vi "Progra 15.vi"() -> ()   [LabVIEW 2011]
uses:
  Control 2.ctl
  <vilib>/express/express arith-compare/Formula/XNode/ExpressFormulaBlockNode.xnode
panel:
  out "Array 2":string[](array[string])
  out "Array":dbl[](array[numeric])
  # "En el arreglo 1 ingresar 5 numeros enteros y luego en el arreglo 2\nescribir si es par o impar cada uno de los numeros"
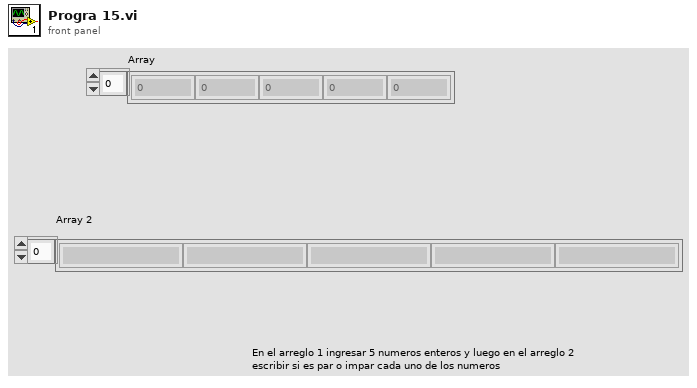
[diagram p1: front panel]
types:
  T1 = typedef "Control 2.ctl" = enum16{"Iniciar Arreglos", "Rellenar Arreglos", "Encontrar ParesImpares", "Final"}
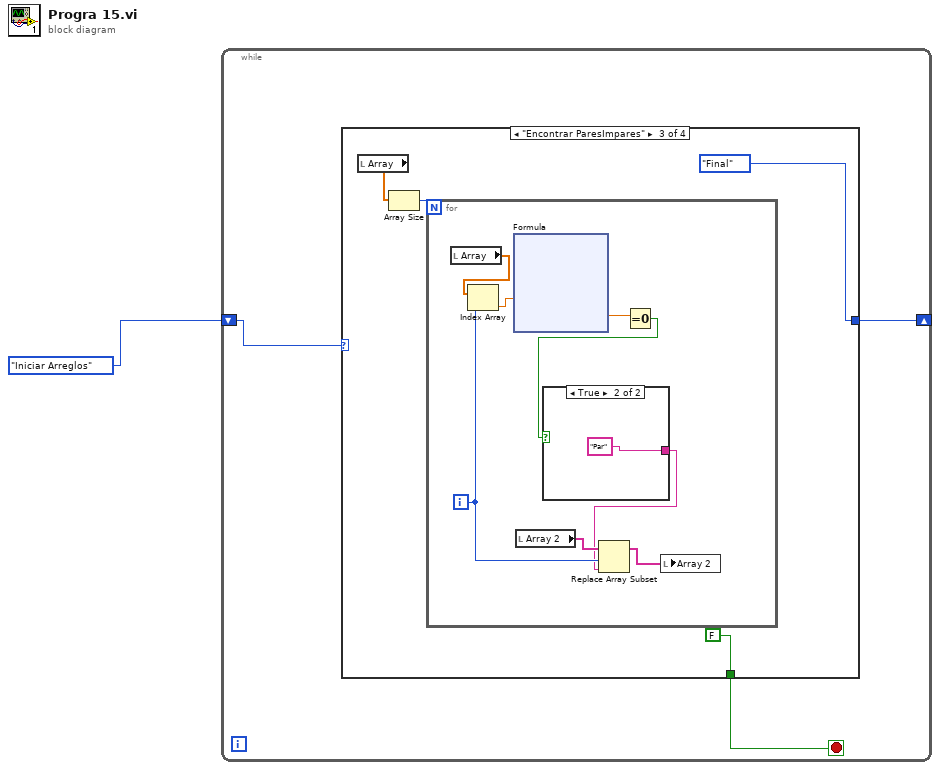
[diagram p0: block diagram]
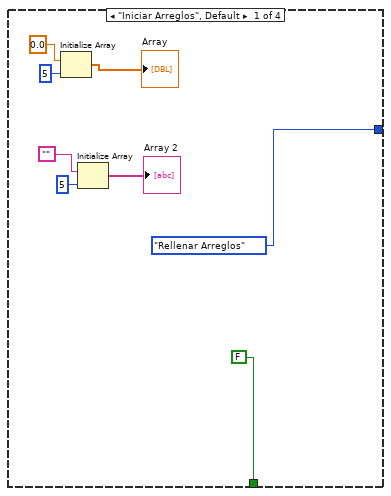
[diagram p2: hidden frame]
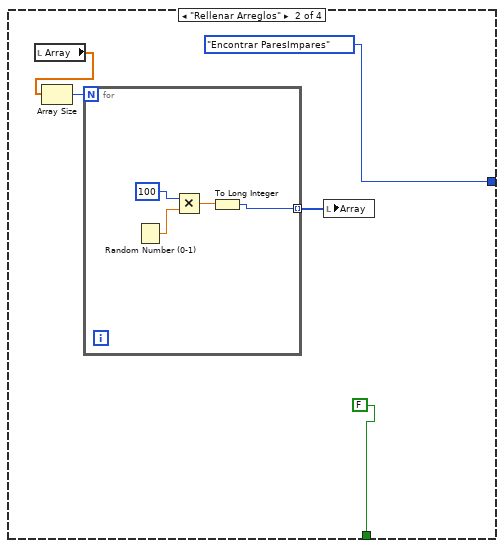
[diagram p3: hidden frame]
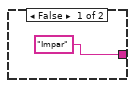
[diagram p4: hidden frame]
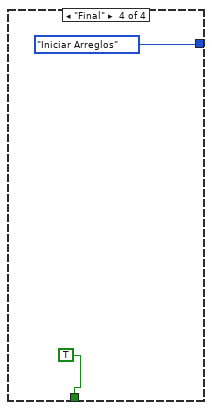
[diagram p5: hidden frame]
diagram:
  n1 = while {
    shift-right: [w2] -> _
    shift-left: Control_2."Iniciar Arreglos" -> [w4]
    stop <- w3 stop-if-true
    n2 = case shown="\"Encontrar ParesImpares\"" w4 {
      tunnel: [FALSE FALSE FALSE TRUE] -> w3
      tunnel: [Control_2."Rellenar Arreglos" Control_2."Encontrar ParesImpares" Control_2."Final" Control_2."Iniciar Arreglos"] -> w2
      frame "Iniciar Arreglos", Default {
        n3 = Initialize Array(0.0 ("element"), 5 ("dimension size")) -> (→"Array":dbl[])
        n4 = Initialize Array("", 5 ("dimension size")) -> (→"Array 2":string[])
      }
      frame "Rellenar Arreglos" {
        n5 = local read "Array"() -> (w17:dbl[])
        n6 = Array Size(array=w17) -> (size(s)=w16:i32)
        n7 = for {
          N: w16 -> [_]
          tunnel: [w18] -> w15 mode=indexing
          n8 = Random Number (0-1)() -> (number: 0 to 1=w20:dbl)
          n9 = Multiply(x=100, y=w20) -> (x*y=w19:dbl)
          n10 = To Long Integer(number=w19) -> (32bit integer=w18:i32)
        }
        n11 = local write "Array"(w15) -> ()
      }
      frame "Encontrar ParesImpares" {
        n12 = local read "Array"() -> (w24:dbl[])
        n13 = Array Size(array=w24) -> (size(s)=w25:i32)
        n14 = for {
          N: w25 -> [_]
          i -> [w28]
          n15 = local read "Array"() -> (w33:dbl[])
          n16 = Index Array(array=w33, index=w28) -> (element=w32:dbl)
          n17 = xnode "Formula"("X1"=w32) -> ("Result"=w31:dbl)  [unwired: 1 in, 1 out]
          n18 = local read "Array 2"() -> (w29:string[])
          n19 = Equal To 0?(x=w31) -> (x = 0?=w30:bool)
          n20 = case shown="True" w30 {
            tunnel: ["Impar" "Par"] -> w27
            frame False {
            }
            frame True {
            }
          }
          n21 = Replace Array Subset(array=w29, new element=w27, index=w28) -> (w26:string[])
          n22 = local write "Array 2"(w26) -> ()
        }
      }
      frame "Final" {
      }
    }
  }
